vi "JIG_RESET_separated.vi"(10 "JIG_RESET":bool, 11 "Mem_mapping in":u16[](array[numeric])) -> (3 "Mem_mapping out":u16[](array[numeric]))   [LabVIEW 2018, in "MB Relay.lvlib"]
uses:
  MB Relay.lvlib
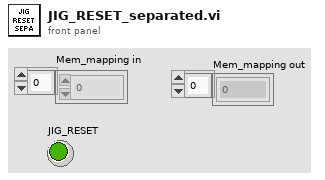
[diagram p1: front panel]
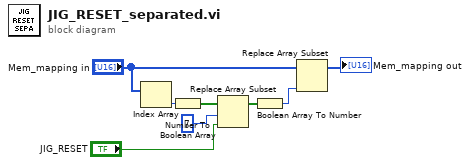
[diagram p0: block diagram]
diagram:
  n1 = Index Array(array="Mem_mapping in") -> (element=w7:u16)  [unwired: 1 in]
  n2 = Number To Boolean Array(number=w7) -> (Boolean array=w8:bool[])
  n3 = Replace Array Subset(array=w8, new element="JIG_RESET", index=7) -> (w4:bool[])
  n4 = Boolean Array To Number(Boolean array=w4) -> (number=w3:u16)
  n5 = Replace Array Subset(array="Mem_mapping in", new element=w3) -> (→"Mem_mapping out":u16[])  [unwired: 1 in]
